vi "Init.vi"(8 "error in (no error)":errorcluster, 10 "Test Tree reference":refnum<vi>, 11 "Test Tree In":refnum<class "Test Tree.lvclass">) -> (0 "error out":errorcluster, 3 "Test Tree Out":refnum<class "Test Tree.lvclass">)   [LabVIEW 2020, in "Test Tree.lvclass"]
uses:
  Test Tree.lvclass
  Test Tree.lvclass/Test Tree.ctl
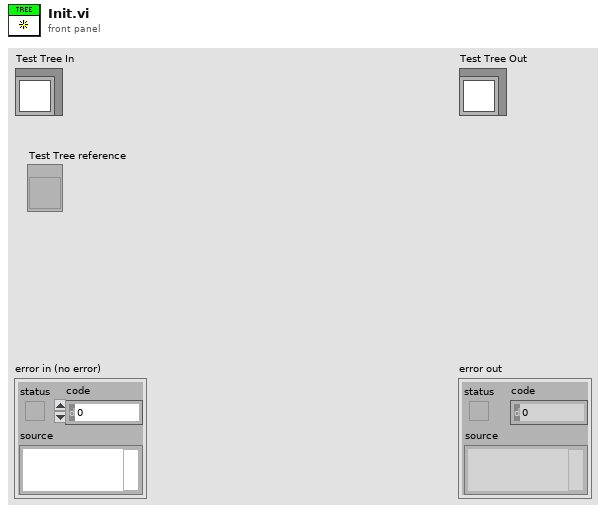
[diagram p1: front panel]
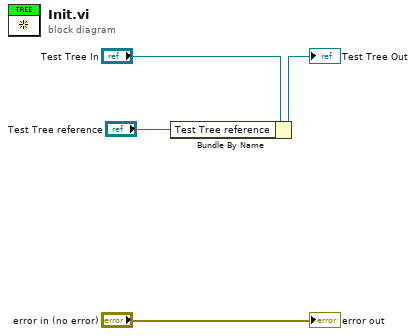
[diagram p0: block diagram]
diagram:
  n1 = Bundle By Name(cluster="Test Tree In", "Test Tree reference"="Test Tree reference") -> (→"Test Tree Out":refnum<class "Test Tree.lvclass">)
  "error out" <- "error in (no error)"
